vi "Teleop.vi"(10 "Match Info":T1={"Autonomous Elapsed Seconds"=0.0, "TeleOp Elapsed Seconds"=0.0, "Disabled Elapsed Seconds"=0.0, "Visited Autonomous"=FALSE, "Visited TeleOp"=FALSE, "Visited Disabled"=FALSE, "Autonomous Settings"={"Autonomous Style"=enum."Independent", "VI Refnum"=refnum}}, 11 "Call Context":T2) -> ()   [LabVIEW 2012]
doc: "This VI is called for each TeleOp packet received from the DS where the robot is not disabled. It is often used to read from the joysticks and update I/O or to update setpoints for timed control loops. It should complete and return within 20 milliseconds or it may miss DS packets."
uses:
  <vilib>/Rock Robotics/WPI/DriverStation/WPI_DriverStationDerivedRobotMode.ctl
  <vilib>/Rock Robotics/WPI/DriverStation/WPI_DriverStationMatch Info.ctl
  Begin/Robot Global Data.vi
  Begin/Global Refnums.vi
  Begin/Global Variables.vi
  <vilib>/Rock Robotics/WPI/Joystick/WPI_JoystickGetSetRefNum.vi
panel:
  out "Numeric 1":dbl(slide) scale=0.0..100.0
  out "Boolean 2":bool
  out "Boolean 1":bool
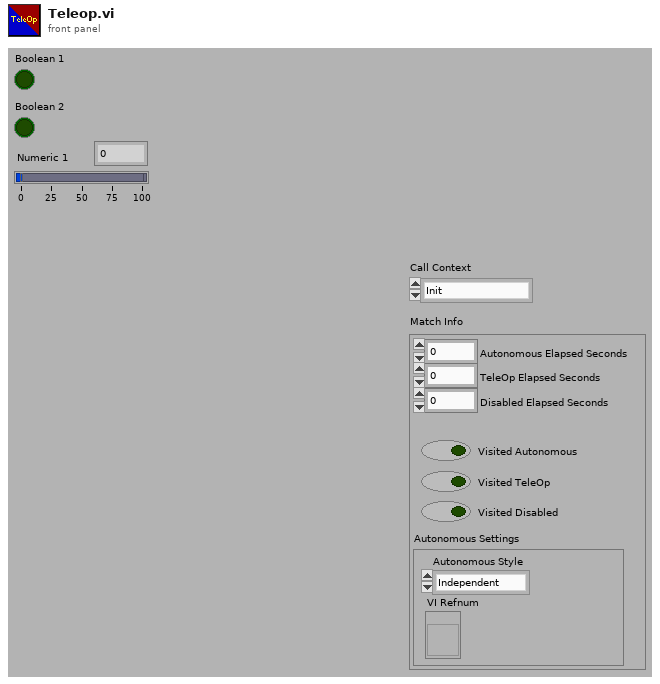
[diagram p1: front panel]
types:
  T1 = typedef "WPI_DriverStationMatch Info.ctl" = cluster{"Autonomous Elapsed Seconds":dbl, "TeleOp Elapsed Seconds":dbl, "Disabled Elapsed Seconds":dbl, "Visited Autonomous":bool, "Visited TeleOp":bool, "Visited Disabled":bool, "Autonomous Settings":cluster{"Autonomous Style":enum16{"Iterative", "Independent"}, "VI Refnum":refnum<vi>}}
  T2 = typedef "WPI_DriverStationDerivedRobotMode.ctl" = enum16{"Init", "Execute", "Stop"}
  T3 = typedef "WPI_JoystickDevRef.ctl" = cluster{"Device":T4}
  T4 = typedef "WPI_JoystickDeviceEnum.ctl" = enum16{"USB 1", "USB 2", "USB 3", "USB 4", "Kinect 1", "Kinect 2"}
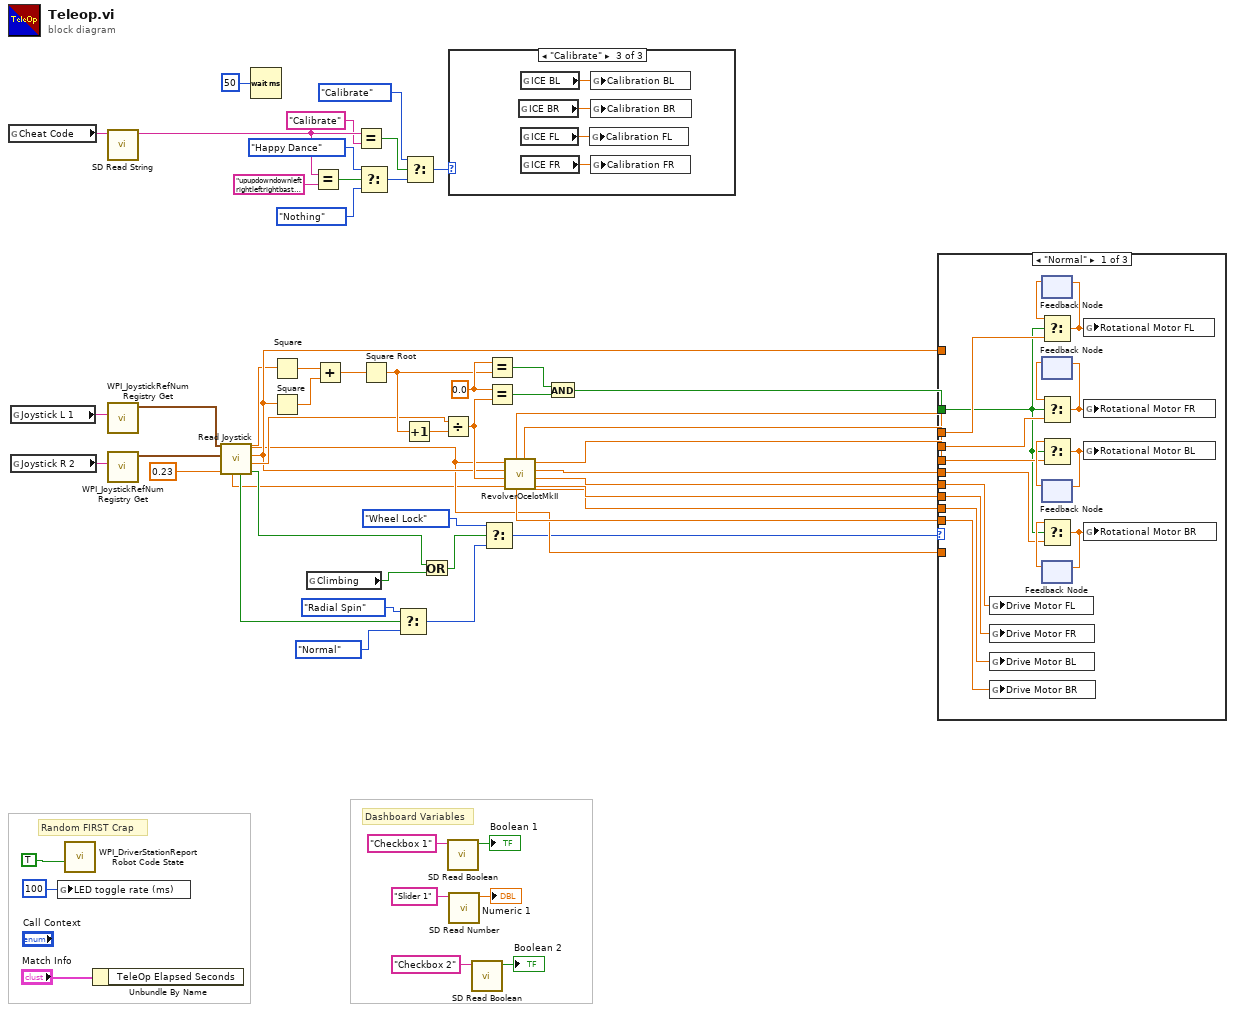
[diagram p0: block diagram]
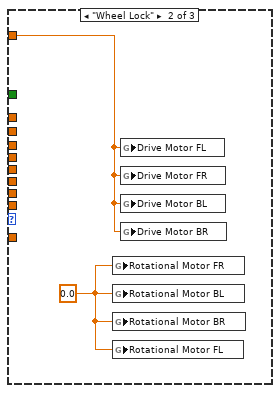
[diagram p2: hidden frame]
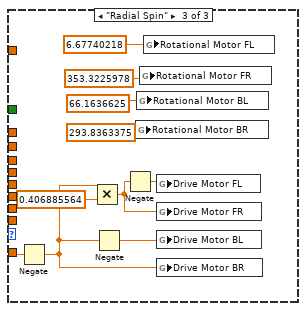
[diagram p3: hidden frame]
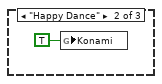
[diagram p5: hidden frame]
diagram:
  w30 = 0.0 ("x")
  # "Dashboard Variables"
  # "Random FIRST Crap"
  n1 = global read "Global Refnums.vi" "Cheat Code"() -> (w47:string)
  n2 = global read "Global Refnums.vi" "Joystick L 1"() -> (w43:string)
  n3 = global read "Global Refnums.vi" "Joystick R 2"() -> (w42:string)
  n4 = global write "Robot Global Data.vi" "LED toggle rate (ms)"(u32 100 ("LED ms toggle rate")) -> ()
  n5 = call <vilib>:"WPI_DriverStationReport Robot Code State.vi"("TeleOp"=TRUE ("Autonomous")) -> ()  [unwired: 10 in, 1 out]
  n6 = Unbundle By Name("Match Info") -> ()  [unwired: 1 out]
  n7 = call <vilib>:"SD Read String.vi"("Name"=w47) -> ("String"=w48:string)  [unwired: 8 in, 2 out]
  n8 = call <vilib>:"WPI_JoystickRefNum Registry Get.vi"("refnum name"=w43) -> ("JoystickDevRef"=w44:T3)  [unwired: 9 in, 1 out]
  n9 = call <vilib>:"WPI_JoystickRefNum Registry Get.vi"("refnum name"=w42) -> ("JoystickDevRef"=w45:T3)  [unwired: 9 in, 1 out]
  n10 = call "Read Joystick.vi"("Joystick Deadbanded Value (default of 0.1)"=0.23, "Joystick R 2 DevRef"=w45, "Joystick L 1 DevRef"=w44) -> ("Wheel Lock"=w6:bool, "Joystick R 2 X Axis"=w9:dbl, "Joystick L 1 Y Axis"=w8:dbl, "Joystick L 1 X Axis"=w7:dbl, "Radial Spin"=w2:bool, "axis 3 (throttle)"=w1:dbl)  [unwired: 3 in]
  n11 = Wait (ms)(milliseconds to wait=u32 50) -> ()  [unwired: 1 out]
  n12 = Square(x=w7) -> (x^2=w36:dbl)
  n13 = Square(x=w8) -> (x^2=w37:dbl)
  n14 = global read "Global Variables.vi" "Climbing"() -> (w4:bool)
  n15 = Equal?(x=w48, y="upupdowndownleftrightleftrightbastart") -> (x = y?=w22:bool)
  n16 = Add(x=w36, y=w37) -> (x+y=w35:dbl)
  n17 = Equal?(x=w48, y="Calibrate") -> (x = y?=w26:bool)
  n18 = Select(t=enum16{"Nothing", "Happy Dance", "Calibrate"}."Happy Dance", s=w22, f=enum16{"Nothing", "Happy Dance", "Calibrate"}."Nothing") -> (s? t:f=w20:enum16{"Nothing", "Happy Dance", "Calibrate"})
  n19 = Square Root(x=w35) -> (sqrt(x)=w28:dbl)
  n20 = Select(t=enum16{"Normal", "Wheel Lock", "Radial Spin"}."Radial Spin", s=w2, f=enum16{"Normal", "Wheel Lock", "Radial Spin"}."Normal") -> (s? t:f=w13:enum16{"Normal", "Wheel Lock", "Radial Spin"})
  n21 = Increment(x=w28) -> (x+1=w29:dbl)
  n22 = Select(t=enum16{"Nothing", "Happy Dance", "Calibrate"}."Calibrate", s=w26, f=w20) -> (s? t:f=w24:enum16{"Nothing", "Happy Dance", "Calibrate"})
  n23 = Or(x=w6, y=w4) -> (x .or. y?=w5:bool)
  n24 = Divide(x=w9, y=w29) -> (x/y=w14:dbl)
  n25 = call <vilib>:"SD Read Boolean.vi"("Name"="Checkbox 1" ("refnum name")) -> ("Boolean"=→"Boolean 1":bool)  [unwired: 8 in, 2 out]
  n26 = case shown="\"Calibrate\"" w24 {
    frame "Nothing", Default {
    }
    frame "Happy Dance" {
      n27 = global write "Global Variables.vi" "Konami"(TRUE) -> ()
    }
    frame "Calibrate" {
      n28 = global read "Global Variables.vi" "ICE BR"() -> (w61:dbl)
      n29 = global read "Global Variables.vi" "ICE BL"() -> (w62:dbl)
      n30 = global read "Global Variables.vi" "ICE FL"() -> (w60:dbl)
      n31 = global read "Global Variables.vi" "ICE FR"() -> (w59:dbl)
      n32 = global write "Global Variables.vi" "Calibration FL"(w60) -> ()
      n33 = global write "Global Variables.vi" "Calibration BL"(w62) -> ()
      n34 = global write "Global Variables.vi" "Calibration BR"(w61) -> ()
      n35 = global write "Global Variables.vi" "Calibration FR"(w59) -> ()
    }
  }
  n36 = call <vilib>:"SD Read Number.vi"("Name"="Slider 1" ("refnum name")) -> ("Numeric"=→"Numeric 1":dbl)  [unwired: 8 in, 2 out]
  n37 = call <vilib>:"SD Read Boolean.vi"("Name"="Checkbox 2" ("refnum name")) -> ("Boolean"=→"Boolean 2":bool)  [unwired: 8 in, 2 out]
  n38 = Select(t=enum16{"Normal", "Wheel Lock", "Radial Spin"}."Wheel Lock", s=w5, f=w13) -> (s? t:f=w3:enum16{"Normal", "Wheel Lock", "Radial Spin"})
  n39 = Equal?(x=w30, y=w28) -> (x = y?=w32:bool)
  n40 = Equal?(x=w30, y=w14) -> (x = y?=w31:bool)
  n41 = call "RevolverOcelotMkII.vi"("Triggers"=w1, "RCW (X2)"=w14, "FWD (Y)"=w8, "STR (X)"=w7) -> ("FRD"=w17:dbl, "FLD"=w18:dbl, "BRS"=w40:dbl, "BLS"=w39:dbl, "BLD"=w16:dbl, "FRS"=w38:dbl, "BRD"=w15:dbl, "FLS"=w34:dbl)
  n42 = And(x=w32, y=w31) -> (x .and. y?=w33:bool)
  n43 = case shown="\"Normal\"" w3 {
    tunnel: w40 -> [w75 _ _]
    tunnel: w39 -> [w74 _ _]
    tunnel: w38 -> [w73 _ _]
    tunnel: w34 -> [w70 _ _]
    tunnel: w33 -> [w67 _ _]
    tunnel: w18 -> [w66 _ _]
    tunnel: w17 -> [w65 _ _]
    tunnel: w16 -> [w64 _ _]
    tunnel: w15 -> [w63 _ _]
    tunnel: w7 -> [_ _ w86]
    tunnel: w8 -> [_ w80 _]
    frame "Normal" {
      n44 = global write "Global Variables.vi" "Drive Motor FL"(w66) -> ()
      n45 = global write "Global Variables.vi" "Drive Motor FR"(w65) -> ()
      n46 = global write "Global Variables.vi" "Drive Motor BL"(w64) -> ()
      n47 = global write "Global Variables.vi" "Drive Motor BR"(w63) -> ()
      n48 = feedback #1() -> (w79:dbl)  [unwired: 1 in]
      n49 = Select(t=w79, s=w67, f=w70) -> (s? t:f=w69:dbl)
      n50 = feedback-in #1(w69) -> ()
      n51 = feedback #2() -> (w78:dbl)  [unwired: 1 in]
      n52 = Select(t=w78, s=w67, f=w73) -> (s? t:f=w72:dbl)
      n53 = feedback-in #2(w72) -> ()
      n54 = feedback #3() -> (w77:dbl)  [unwired: 1 in]
      n55 = Select(t=w77, s=w67, f=w74) -> (s? t:f=w71:dbl)
      n56 = feedback-in #3(w71) -> ()
      n57 = feedback #4() -> (w76:dbl)  [unwired: 1 in]
      n58 = Select(t=w76, s=w67, f=w75) -> (s? t:f=w68:dbl)
      n59 = feedback-in #4(w68) -> ()
      n60 = global write "Global Variables.vi" "Rotational Motor FL"(w69) -> ()
      n61 = global write "Global Variables.vi" "Rotational Motor FR"(w72) -> ()
      n62 = global write "Global Variables.vi" "Rotational Motor BL"(w71) -> ()
      n63 = global write "Global Variables.vi" "Rotational Motor BR"(w68) -> ()
    }
    frame "Wheel Lock" {
      w81 = 0.0
      n64 = global write "Global Variables.vi" "Rotational Motor FR"(w81) -> ()
      n65 = global write "Global Variables.vi" "Rotational Motor BL"(w81) -> ()
      n66 = global write "Global Variables.vi" "Rotational Motor BR"(w81) -> ()
      n67 = global write "Global Variables.vi" "Rotational Motor FL"(w81) -> ()
      n68 = global write "Global Variables.vi" "Drive Motor FL"(w80) -> ()
      n69 = global write "Global Variables.vi" "Drive Motor FR"(w80) -> ()
      n70 = global write "Global Variables.vi" "Drive Motor BL"(w80) -> ()
      n71 = global write "Global Variables.vi" "Drive Motor BR"(w80) -> ()
    }
    frame "Radial Spin" {
      n72 = Negate(x=w86) -> (-x=w82:dbl)
      n73 = Multiply(x=w82, y=0.406885564) -> (x*y=w85:dbl)
      n74 = Negate(x=w82) -> (-x=w83:dbl)
      n75 = Negate(x=w85) -> (-x=w84:dbl)
      n76 = global write "Global Variables.vi" "Rotational Motor BR"(293.8363375) -> ()
      n77 = global write "Global Variables.vi" "Rotational Motor BL"(66.1636625) -> ()
      n78 = global write "Global Variables.vi" "Rotational Motor FR"(353.3225978) -> ()
      n79 = global write "Global Variables.vi" "Rotational Motor FL"(6.67740218) -> ()
      n80 = global write "Global Variables.vi" "Drive Motor FL"(w84) -> ()
      n81 = global write "Global Variables.vi" "Drive Motor FR"(w85) -> ()
      n82 = global write "Global Variables.vi" "Drive Motor BL"(w83) -> ()
      n83 = global write "Global Variables.vi" "Drive Motor BR"(w82) -> ()
    }
  }
